vi "Handle Command.vi"(8 "error in (no error)":errorcluster, 9 "Data":variant, 10 "Command":string, 11 "Instrument.VRM in":refnum<class "Instrument.OxfordVRM.lvclass">) -> (0 "error out":errorcluster, 1 "Processed Data":variant, 2 "Command":string, 3 "Instrument.VRM out":refnum<class "Instrument.OxfordVRM.lvclass">)   [LabVIEW 2019, in "Instrument.OxfordVRM.lvclass"]
uses:
  Instrument.OxfordVRM.lvclass
  Typedefs/Instrument.VRM.publicCommands-enum.ctl
  Typedefs/Instrument.VRM.protectedCommands-enum.ctl
  <userlib>/LevyLab/Instrument Framework/Instrument Types/Cryostat/Typedefs/getMagnet--cluster.ctl
  <userlib>/LevyLab/Instrument Framework/Instrument Types/Cryostat/Typedefs/Magnet Axis--Enum.ctl
  Instrument.OxfordVRM.lvclass/Instrument.OxfordVRM.ctl
  <userlib>/LevyLab/Instrument Framework/Instrument Types/Cryostat/Typedefs/getMagnetVector--cluster.ctl
  <userlib>/LevyLab/Instrument Framework/Instrument Types/Cryostat/Typedefs/setMagnet--cluster.ctl
  <userlib>/LevyLab/Instrument Framework/Instrument Types/Cryostat/Typedefs/Magnet Mode--Enum.ctl
  <userlib>/LevyLab/Instrument Framework/Instrument Types/Cryostat/Typedefs/setMagnetVector--cluster.ctl
  Typedefs/Instrument.VRM.GetTarget--cluster.ctl
  Typedefs/Instrument.VRM.GetField--cluster.ctl
  Typedefs/Instrument.VRM.GetStatus--cluster.ctl
  94f56870-fe0a-4d8a-afd3-baf115ad0e40.vi
  f1f2bbf0-5438-4127-94f1-d54331c0660a.vi
  26570751-a93b-4058-b2c8-e985c8811ccf.vi
  803d4c64-5e05-4ab7-ab6e-37972034c23e.vi
  29715b08-e5f4-4bfa-ba7c-dac6c161a3e8.vi
  954400c7-22f7-4d30-ae7e-d16b29314bbb.vi
  94f56870-fe0a-4d8a-afd3-baf115ad0e40.vi/68bea999-b910-4e00-8aa8-3861bc3a0e24.vi
  94f56870-fe0a-4d8a-afd3-baf115ad0e40.vi/a1666832-1ce1-4593-9a1c-3d97967ebe0c.vi
  f1f2bbf0-5438-4127-94f1-d54331c0660a.vi/4f757dbd-0e49-48ce-aff2-3d2fbadf6e86.vi
  f1f2bbf0-5438-4127-94f1-d54331c0660a.vi/be56346c-dc68-47fb-b1ad-49b939db02a3.vi
  29715b08-e5f4-4bfa-ba7c-dac6c161a3e8.vi/c53687d8-82a3-4c5e-b648-4a23dc0e4095.vi
  29715b08-e5f4-4bfa-ba7c-dac6c161a3e8.vi/86ccb06f-b5fd-47f0-a745-ba091c7f7fa7.vi
  954400c7-22f7-4d30-ae7e-d16b29314bbb.vi/822d43cd-0bc4-4130-8b91-306a3f6f2199.vi
  954400c7-22f7-4d30-ae7e-d16b29314bbb.vi/a176c4a9-2bca-48b6-9155-da156fdf6f77.vi
  <vilib>/Utility/Data Type/Get Type Information.vi
  <vilib>/JDP Science/JSONtext/JSON text to Variant.vi
  <vilib>/JDP Science/JSONtext/Variant to JSON Text.vi
  <vilib>/JDP Science/JSONtext/LVClass Serializer/JSONtext LVClass Serializer.lvclass
  <userlib>/LevyLab/Instrument Framework/Instrument Types/Cryostat/Instrument.Cryostat.lvclass
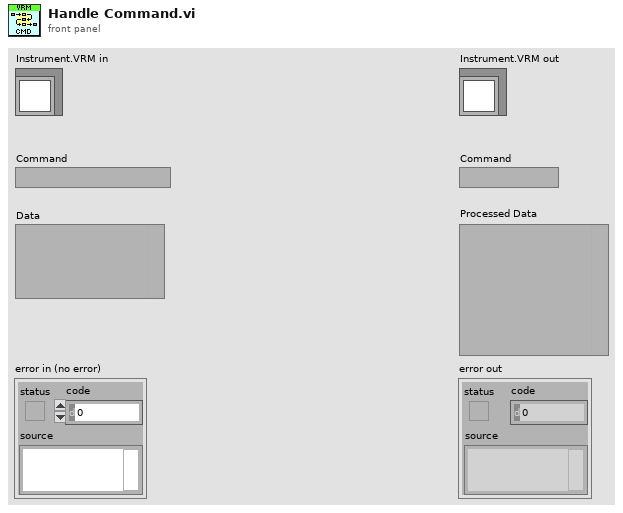
[diagram p1: front panel]
types:
  T1 = typedef "Instrument.OxfordVRM.lvclass/Instrument.VRM.protectedCommands-enum.ctl" = enum16{"Hold", "RampToSet", "RampToZero", "Clamp", "SetTarget", "GetStatus", "GetTarget", "GetField", "setSequenceStatus"}
  T2 = typedef "Instrument.OxfordVRM.lvclass/Instrument.VRM.publicCommands-enum.ctl" = enum16{"setMagnet", "setMagnetVector", "getMagnet", "getMagnetVector", "getMagnetTarget", "getMagnetVectorTarget"}
  T3 = typedef "Instrument.Cryostat.lvclass/Magnet Axis--Enum.ctl" = enum16{"X", "Y", "Z"}
  T4 = typedef "Instrument.Cryostat.lvclass/getMagnet--cluster.ctl" = cluster{"field":dbl, "status":string, "finished":bool}
  T5 = typedef "Instrument.Cryostat.lvclass/getMagnetVector--cluster.ctl" = cluster{"field":dbl[], "status":string, "finished":bool}
  T6 = typedef "Instrument.Cryostat.lvclass/setMagnet--cluster.ctl" = cluster{"field":dbl, "rate":dbl, "axis":T3, "mode":T7}
  T7 = typedef "Instrument.Cryostat.lvclass/Magnet Mode--Enum.ctl" = enum16{"Persistent", "Driven"}
  T8 = typedef "Instrument.Cryostat.lvclass/setMagnetVector--cluster.ctl" = cluster{"field":dbl[], "rate":dbl}
  T9 = typedef "Instrument.OxfordVRM.lvclass/Instrument.VRM.GetTarget--cluster.ctl" = cluster{"field":dbl[], "rate":dbl[]}
  T10 = typedef "Instrument.OxfordVRM.lvclass/Instrument.VRM.GetField--cluster.ctl" = cluster{"field":dbl[]}
  T11 = typedef "Instrument.OxfordVRM.lvclass/Instrument.VRM.GetStatus--cluster.ctl" = cluster{"Status":string[]}
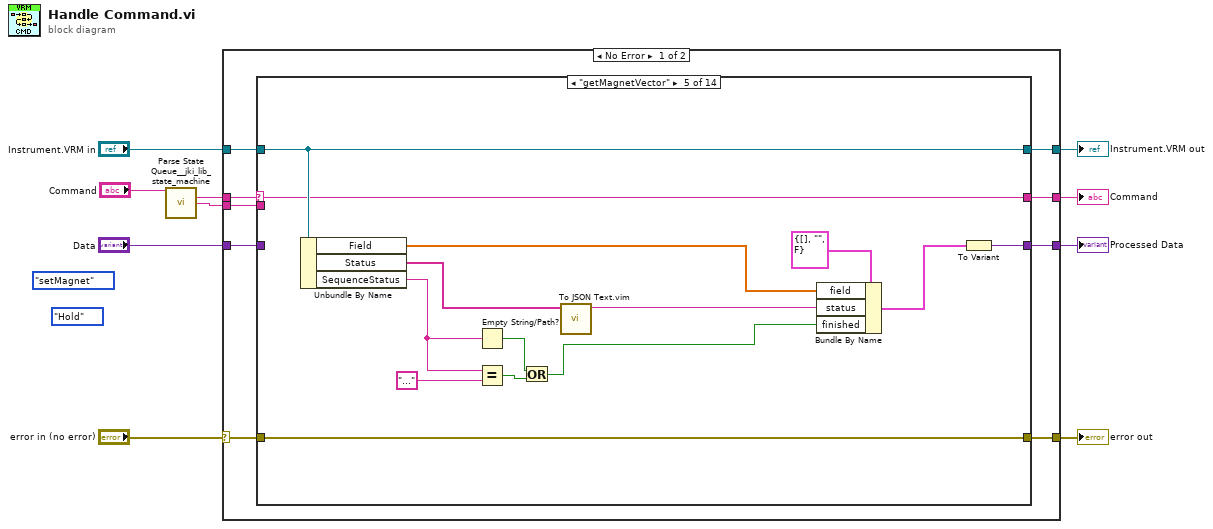
[diagram p0: block diagram]
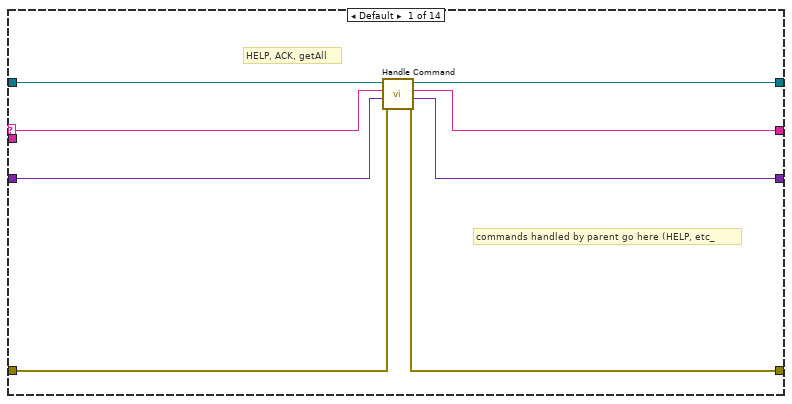
[diagram p2: hidden frame]
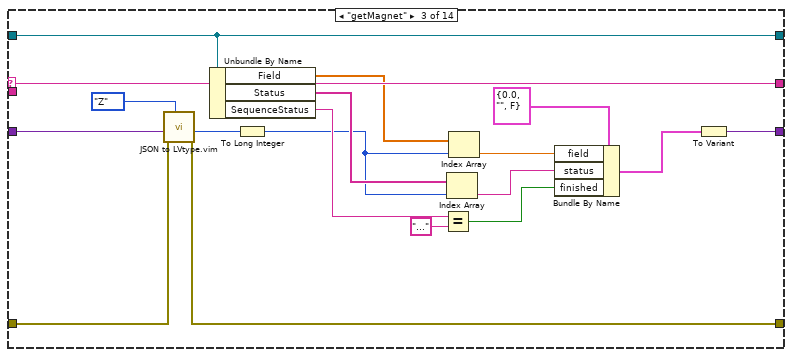
[diagram p4: hidden frame]
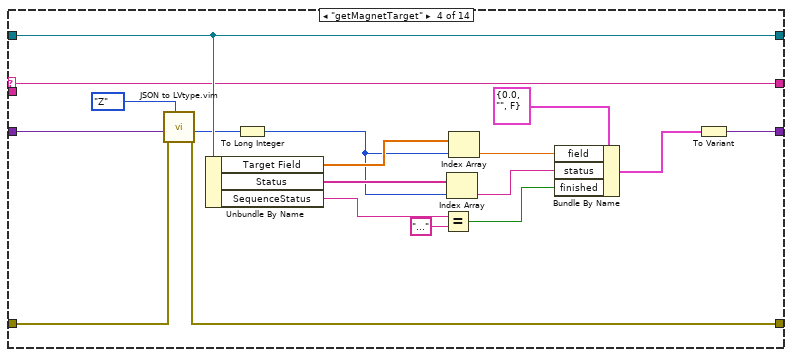
[diagram p5: hidden frame]
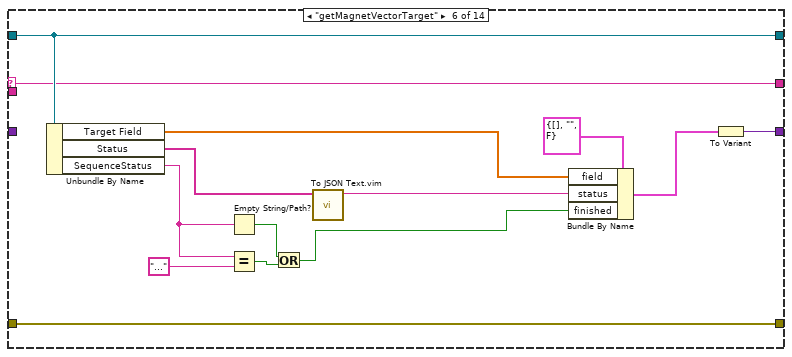
[diagram p6: hidden frame]
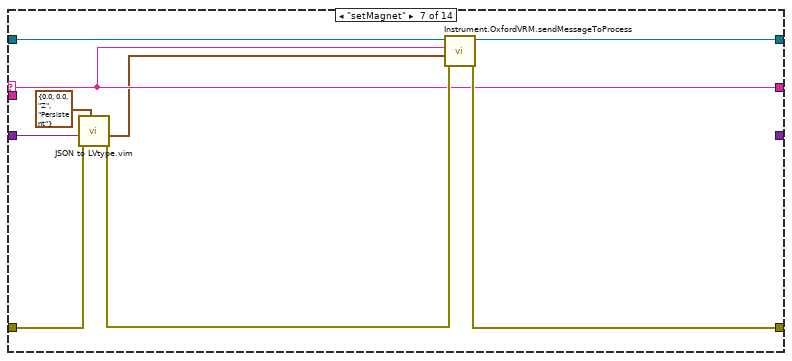
[diagram p7: hidden frame]
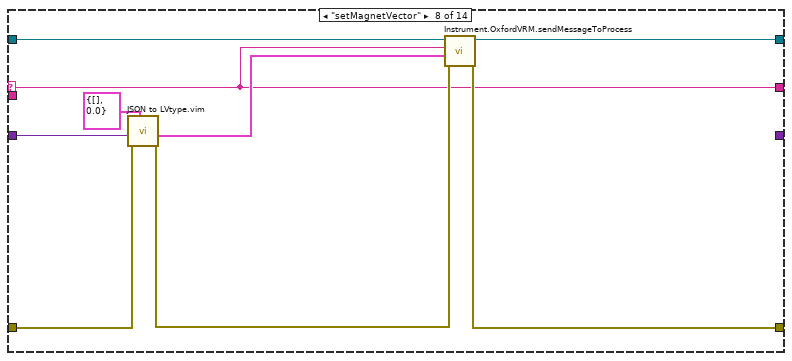
[diagram p8: hidden frame]
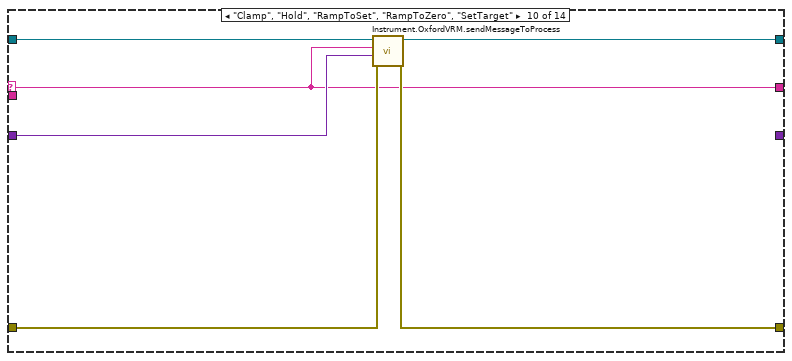
[diagram p10: hidden frame]
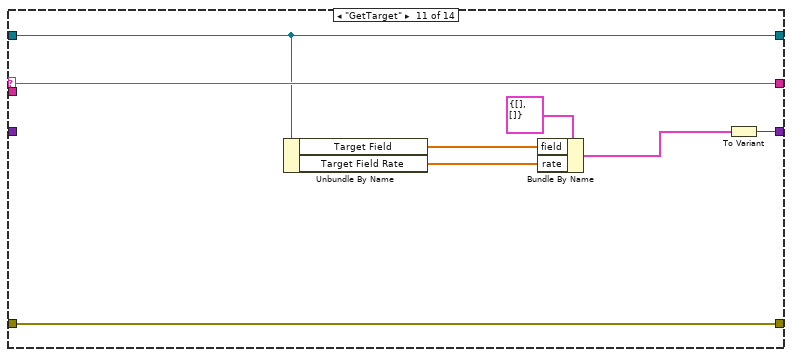
[diagram p11: hidden frame]
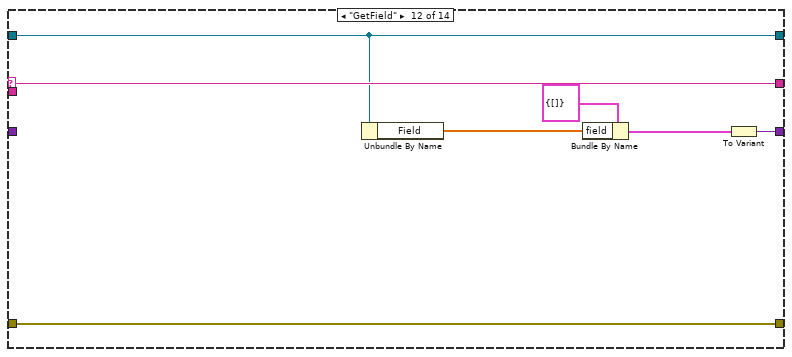
[diagram p12: hidden frame]
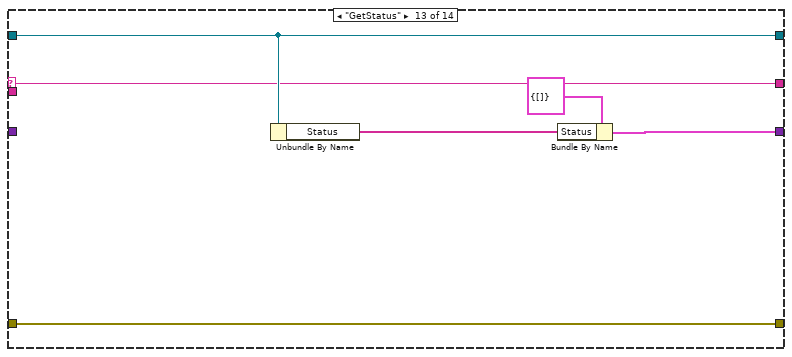
[diagram p13: hidden frame]
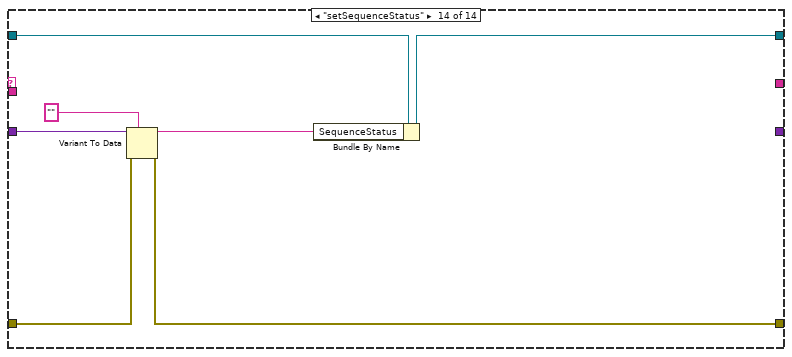
[diagram p14: hidden frame]
diagram:
  (unwired) Instrument.VRM.protectedCommands-enum."Hold" ("protectedCommands")
  (unwired) Instrument.VRM.publicCommands-enum."setMagnet" ("Commands")
  n1 = call <vilib>:"Parse State Queue__jki_lib_state_machine.vi"("State Queue"="Command") -> ("Current State"=w2:string, "Arguments"=w1:string)  [unwired: 12 in, 1 out]
  n2 = case shown="No Error" "error in (no error)" {
    selector: "error in (no error)" -> [w12 w148]
    tunnel: [w15 w148] -> w10
    tunnel: [w19 _] -> w9
    tunnel: [w18 _] -> w8
    tunnel: [w17 w149] -> w7
    tunnel: "Data" -> [w11 _]
    tunnel: w2 -> [w13 _]
    tunnel: "Instrument.VRM in" -> [w16 w149]
    tunnel: w1 -> [w14 _]
    frame No Error {
      n3 = case shown="\"getMagnetVector\"" w13 {
        selector: w13 -> [w20 _ w46 w64 w78 w92 w95 w103 _ w114 w126 w133 w139 _]
        tunnel: [w22 _ w31 w50 w73 w87 _ _ _ _ w127 w134 w136 _] -> w19
        tunnel: [w27 _ w46 w64 w78 w92 w95 w103 _ w114 w126 w133 w139 _] -> w18
        tunnel: [w26 w29 w47 w65 w79 w93 w101 w110 w113 w116 w120 w129 w140 w141] -> w17
        tunnel: w11 -> [w21 _ w43 w61 _ _ w99 w107 _ w115 _ _ _ w147]
        tunnel: w16 -> [w25 w29 w47 w65 w79 w93 w102 w111 w113 w119 w120 w129 w140 w144]
        tunnel: w12 -> [w24 w28 w44 w62 w77 w91 w97 w106 w112 w118 w125 w132 w135 w145]
        tunnel: [w23 w28 w45 w63 w77 w91 w100 w109 w112 w117 w125 w132 w135 w142] -> w15
        tunnel: w14 -> [_ _ _ _ _ _ _ _ _ _ _ _ _ _]
        frame Default {
          # "HELP, ACK, getAll"
          # "commands handled by parent go here (HELP, etc_"
          n4 = call-parent "Handle Command.vi"("error in (no error)"=w24, "params in"=w21, "command"=w20, "Instrument in"=w25) -> ("error out"=w23:errorcluster, "processed data"=w22:variant, "command out"=w27:string, "Instrument out"=w26:refnum<class "Instrument.OxfordVRM.lvclass">)  [unwired: 4 in]
        }
        frame "--- Public Methods ---" {
        }
        frame "getMagnet" {
          n5 = call "JSON to LVtype.vim"("type"=Magnet_Axis--Enum."Z" ("Axis"), "error in (no error)"=w44, "JSON Data in"=w43) -> ("error out"=w45:errorcluster, "Data out"=w37:T3)  [unwired: 7 in]
          n6 = Unbundle By Name(w47) -> ("Field"=w40:dbl[], "Status"=w38:string[], "SequenceStatus"=w35:string)
          n7 = To Long Integer(number=w37) -> (32bit integer=w30:i32)
          n8 = Equal?(x=w35, y="...") -> (x = y?=w33:bool)
          n9 = Index Array(array=w38, index=w30) -> (element=w36:string)
          n10 = Index Array(array=w40, index=w30) -> (element=w39:dbl)
          n11 = Bundle By Name(cluster=T4 {"field"=0.0, "status"="", "finished"=FALSE} ("getMagnet"), "field"=w39, "status"=w36, "finished"=w33) -> (w32:T4)
          n12 = To Variant(anything=w32) -> (Variant=w31:variant)
        }
        frame "getMagnetTarget" {
          n13 = call "JSON to LVtype.vim"("type"=Magnet_Axis--Enum."Z" ("Axis"), "error in (no error)"=w62, "JSON Data in"=w61) -> ("error out"=w63:errorcluster, "Data out"=w55:T3)  [unwired: 7 in]
          n14 = Unbundle By Name(w65) -> ("Target Field"=w58:dbl[], "Status"=w56:string[], "SequenceStatus"=w48:string)
          n15 = To Long Integer(number=w55) -> (32bit integer=w49:i32)
          n16 = Equal?(x=w48, y="...") -> (x = y?=w52:bool)
          n17 = Index Array(array=w56, index=w49) -> (element=w54:string)
          n18 = Index Array(array=w58, index=w49) -> (element=w57:dbl)
          n19 = Bundle By Name(cluster=T4 {"field"=0.0, "status"="", "finished"=FALSE} ("getMagnet"), "field"=w57, "status"=w54, "finished"=w52) -> (w51:T4)
          n20 = To Variant(anything=w51) -> (Variant=w50:variant)
        }
        frame "getMagnetVector" {
          n21 = Unbundle By Name(w79) -> ("Field"=w72:dbl[], "Status"=w71:string[], "SequenceStatus"=w68:string)
          n22 = Empty String/Path?(string/path=w68) -> (empty?=w67:bool)
          n23 = Equal?(x=w68, y="...") -> (x = y?=w66:bool)
          n24 = Or(x=w67, y=w66) -> (x .or. y?=w69:bool)
          n25 = call "To JSON Text.vim"("Anything"=w71) -> ("<JSON>"=w70:string)  [unwired: 9 in, 1 out]
          n26 = Bundle By Name(cluster=T5 {"field"=[], "status"="", "finished"=FALSE} ("getMagnet"), "field"=w72, "status"=w70, "finished"=w69) -> (w74:T5)
          n27 = To Variant(anything=w74) -> (Variant=w73:variant)
        }
        frame "getMagnetVectorTarget" {
          n28 = Unbundle By Name(w93) -> ("Target Field"=w86:dbl[], "Status"=w85:string[], "SequenceStatus"=w82:string)
          n29 = Empty String/Path?(string/path=w82) -> (empty?=w81:bool)
          n30 = Equal?(x=w82, y="...") -> (x = y?=w80:bool)
          n31 = Or(x=w81, y=w80) -> (x .or. y?=w83:bool)
          n32 = call "To JSON Text.vim"("Anything"=w85) -> ("<JSON>"=w84:string)  [unwired: 9 in, 1 out]
          n33 = Bundle By Name(cluster=T5 {"field"=[], "status"="", "finished"=FALSE} ("getMagnet"), "field"=w86, "status"=w84, "finished"=w83) -> (w88:T5)
          n34 = To Variant(anything=w88) -> (Variant=w87:variant)
        }
        frame "setMagnet" {
          n35 = call "JSON to LVtype.vim"("type"=T6 {"field"=0.0, "rate"=0.0, "axis"=enum."Z", "mode"=enum."Persistent"} ("setMagnet"), "error in (no error)"=w97, "JSON Data in"=w99) -> ("error out"=w96:errorcluster, "Data out"=w94:T6)  [unwired: 7 in]
          n36 = call "Instrument.OxfordVRM.sendMessageToProcess.vi"("error in (no error)"=w96, "Data"=w94, "Command"=w95, "Instrument.Oxford1820"=w102) -> ("error out"=w100:errorcluster, "Instrument.Oxford1820 out"=w101:refnum<class "Instrument.OxfordVRM.lvclass">)  [unwired: 6 in]
        }
        frame "setMagnetVector" {
          n37 = call "JSON to LVtype.vim"("type"=T8 {"field"=[], "rate"=0.0} ("setMagnet"), "error in (no error)"=w106, "JSON Data in"=w107) -> ("error out"=w105:errorcluster, "Data out"=w104:T8)  [unwired: 7 in]
          n38 = call "Instrument.OxfordVRM.sendMessageToProcess.vi"("error in (no error)"=w105, "Data"=w104, "Command"=w103, "Instrument.Oxford1820"=w111) -> ("error out"=w109:errorcluster, "Instrument.Oxford1820 out"=w110:refnum<class "Instrument.OxfordVRM.lvclass">)  [unwired: 6 in]
        }
        frame "--- Protected Methods ---" {
        }
        frame "Clamp", "Hold", "RampToSet", "RampToZero", "SetTarget" {
          n39 = call "Instrument.OxfordVRM.sendMessageToProcess.vi"("error in (no error)"=w118, "Data"=w115, "Command"=w114, "Instrument.Oxford1820"=w119) -> ("error out"=w117:errorcluster, "Instrument.Oxford1820 out"=w116:refnum<class "Instrument.OxfordVRM.lvclass">)  [unwired: 6 in]
        }
        frame "GetTarget" {
          n40 = Unbundle By Name(w120) -> ("Target Field"=w123:dbl[], "Target Field Rate"=w122:dbl[])
          n41 = Bundle By Name(cluster=T9 {"field"=[], "rate"=[]} ("GetTarget"), "field"=w123, "rate"=w122) -> (w121:T9)
          n42 = To Variant(anything=w121) -> (Variant=w127:variant)
        }
        frame "GetField" {
          n43 = Unbundle By Name(w129) -> ("Field"=w131:dbl[])
          n44 = Bundle By Name(cluster=T10 {"field"=[]} ("GetField"), "field"=w131) -> (w130:T10)
          n45 = To Variant(anything=w130) -> (Variant=w134:variant)
        }
        frame "GetStatus" {
          n46 = Unbundle By Name(w140) -> ("Status"=w137:string[])
          n47 = Bundle By Name(cluster=T11 {"Status"=[]} ("GetStatus"), "Status"=w137) -> (w136:T11)
        }
        frame "setSequenceStatus" {
          n48 = Variant To Data(error in=w145, type="", Variant=w147) -> (data=w143:string, error out=w142:errorcluster)
          n49 = Bundle By Name(cluster=w144, "SequenceStatus"=w143) -> (w141:refnum<class "Instrument.OxfordVRM.lvclass">)
        }
      }
    }
    frame Error {
    }
  }
  "error out" <- w10
  "Instrument.VRM out" <- w7
  "Processed Data" <- w9
  "Command" <- w8
